vi "VoltageScanSaveFile.vi"(0 "Path":path, 2 "Stop":dbl, 3 "StepSize/V":dbl, 4 "wait for KepCo":u32, 9 "array":dbl[][](array[numeric])) -> (14 "Filename Out":path, 19 "error out":errorcluster)   [LabVIEW 2014]
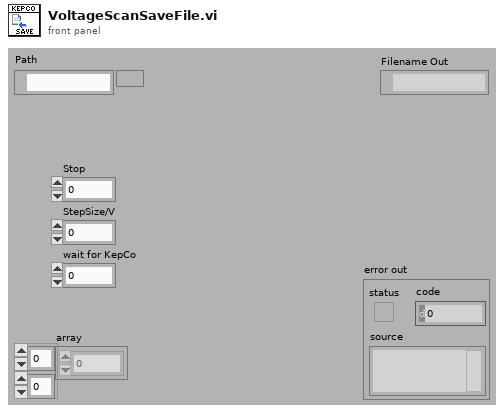
[diagram p1: front panel]
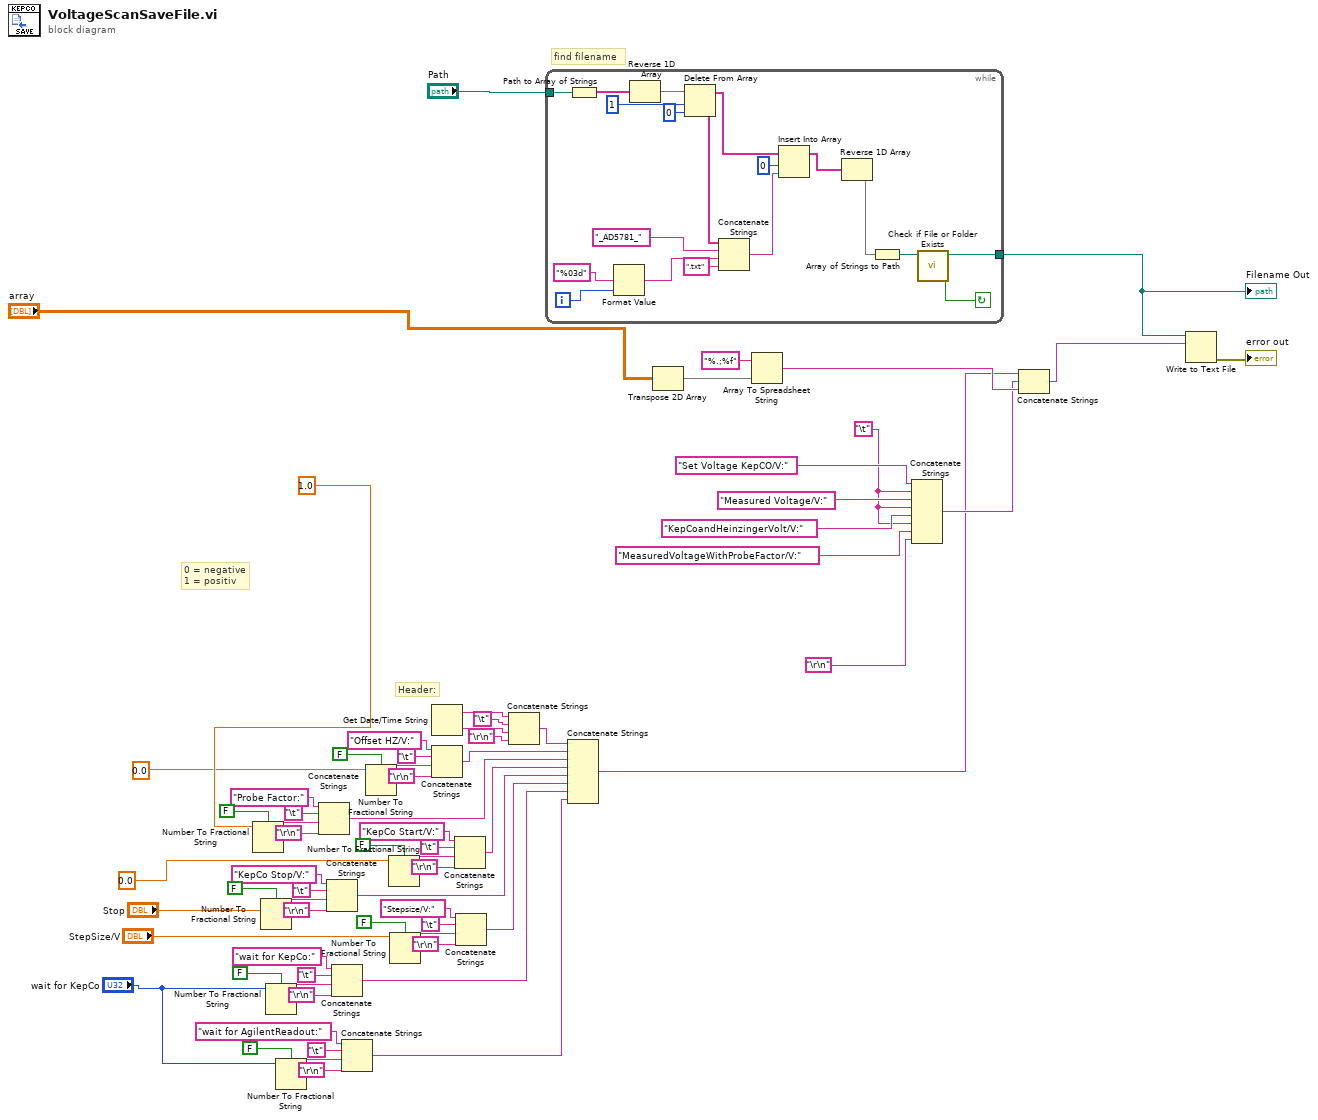
[diagram p0: block diagram]
diagram:
  w59 = "\t"
  # "Header:"
  # "0 = negative\n1 = positiv"
  # "find filename"
  n1 = Number To Fractional String(use system decimal point (T)=FALSE, number=1.0 ("ProbeFactor")) -> (F-format string=w41:string)  [unwired: 2 in]
  n2 = Number To Fractional String(use system decimal point (T)=FALSE, number="Stop") -> (F-format string=w28:string)  [unwired: 2 in]
  n3 = Number To Fractional String(use system decimal point (T)=FALSE, number="wait for KepCo") -> (F-format string=w16:string)  [unwired: 2 in]
  n4 = Number To Fractional String(use system decimal point (T)=FALSE, number="wait for KepCo") -> (F-format string=w9:string)  [unwired: 2 in]
  n5 = Concatenate Strings("Probe Factor:" ("string"), "\t", w41, "\r\n") -> (w38:string)
  n6 = Concatenate Strings("KepCo Stop/V:" ("string"), "\t", w28, "\r\n") -> (w26:string)
  n7 = Concatenate Strings("wait for KepCo:" ("string"), "\t", w16, "\r\n") -> (w14:string)
  n8 = Concatenate Strings("wait for AgilentReadout:" ("string"), "\t", w9, "\r\n") -> (w7:string)
  n9 = Number To Fractional String(use system decimal point (T)=FALSE, number=0.0) -> (F-format string=w53:string)  [unwired: 2 in]
  n10 = Number To Fractional String(use system decimal point (T)=FALSE, number=0.0 ("Start/V")) -> (F-format string=w34:string)  [unwired: 2 in]
  n11 = Number To Fractional String(use system decimal point (T)=FALSE, number="StepSize/V") -> (F-format string=w22:string)  [unwired: 2 in]
  n12 = Get Date/Time String() -> (date string=w50:string, time string=w49:string)  [unwired: 3 in]
  n13 = Concatenate Strings("Offset HZ/V:" ("string"), "\t", w53, "\r\n") -> (w51:string)
  n14 = Concatenate Strings("KepCo Start/V:" ("string"), "\t", w34, "\r\n") -> (w32:string)
  n15 = Concatenate Strings("Stepsize/V:" ("string"), "\t", w22, "\r\n") -> (w20:string)
  n16 = Concatenate Strings(w50, "\t", w49, "\r\n") -> (w46:string)
  n17 = while {
    tunnel: [w86] -> w68
    tunnel: "Path" -> [w70]
    i -> [w73]
    stop <- w87 continue-if-true
    n18 = Path to Array of Strings(0:w70) -> (2:w84:string[])  [unwired: 1 out]
    n19 = Format Value(format string="%03d", value (0)=w73) -> (output string=w71:string)  [unwired: 1 in]
    n20 = Reverse 1D Array(array=w84) -> (reversed array=w83:string[])
    n21 = Delete From Array(array=w83, length=1, index=0) -> (deleted portion=w74:string[], array with subset deleted=w79:string[])
    n22 = Concatenate Strings(w74, "_AD5781_", w71, ".txt" ("string")) -> (w78:string)
    n23 = Insert Into Array(array=w79, index=0, new element=w78) -> (w76:string[])
    n24 = Reverse 1D Array(array=w76) -> (reversed array=w75:string[])
    n25 = Array of Strings to Path(0:w75) -> (2:w81:path)  [unwired: 1 in]
    n26 = call <vilib>:"Check if File or Folder Exists.vi"("path"=w81) -> ("file or folder exists?"=w87:bool, "dup path"=w86:path)  [unwired: 8 in, 1 out]
  }
  "Filename Out" <- w68
  n27 = Concatenate Strings(w46, w51, w38, w32, w26, w20, w14, w7) -> (w45:string)
  n28 = Transpose 2D Array(2D array="array") -> (transposed array=w13:dbl[][])
  n29 = Array To Spreadsheet String(array=w13, 3:"%.;%f" ("format string")) -> (spreadsheet string=w65:string)  [unwired: 1 in]
  n30 = Concatenate Strings("Set Voltage KepCO/V:" ("string"), w59, "Measured Voltage/V:" ("string"), w59, "KepCoandHeinzingerVolt/V:" ("string"), w59, "MeasuredVoltageWithProbeFactor/V:" ("string"), "\r\n") -> (w61:string)
  n31 = Concatenate Strings(w45, w61, w65) -> (w64:string)
  n32 = Write to Text File(file (use dialog)=w68, text=w64) -> (error out=→"error out":errorcluster)  [unwired: 2 in, 2 out]
